vi "Create All Message Queues.vi"(8 "error in (no error)":errorcluster) -> (0 "error out":errorcluster, 3 "Message Queues out":T1)   [LabVIEW 2021, in "Message Queue.lvlib"]
doc: "This VI creates and initializes all the message queues for your application. If your application requires more than one message queue, right-click the \"Message Queues\" constant above and select Open Type Def. Add the new Message Queue(s) to the type definition, then initialize them in this VI."
uses:
  Message Queue.lvlib
  All Message Queues.ctl
  Message Cluster.ctl
  Enqueue Message (Single).vi
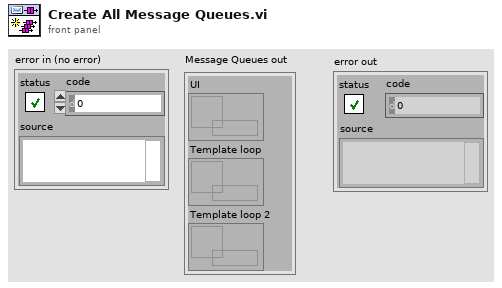
[diagram p1: front panel]
types:
  T1 = typedef "Message Queue.lvlib/All Message Queues.ctl" = cluster{"UI":refnum<queue>, "Template loop":refnum<queue>, "Template loop 2":refnum<queue>}
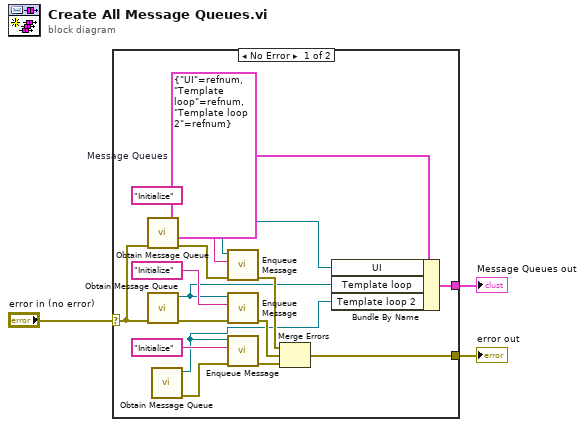
[diagram p0: block diagram]
diagram:
  n1 = case shown="No Error" "error in (no error)" {
    selector: "error in (no error)" -> [w8 w20]
    tunnel: [w10 w20] -> w3
    tunnel: [w18 _] -> w2
    frame No Error {
      w12 = T1 {"UI"=refnum, "Template loop"=refnum, "Template loop 2"=refnum}  # Message Queues
      n2 = call "Obtain Message Queue.vi"("error in (no error)"=w8) -> ("error out"=w17:errorcluster, "Message Queue"=w15:refnum<queue>)  [unwired: 9 in]
      n3 = call "Obtain Message Queue.vi"("error in (no error)"=w8) -> ("error out"=w14:errorcluster, "Message Queue"=w11:refnum<queue>)  [unwired: 9 in]
      n4 = call "Obtain Message Queue.vi"() -> ("error out"=w7:errorcluster, "Message Queue"=w4:refnum<queue>)  [unwired: 10 in]
      n5 = call-poly "Enqueue Message.vi"("error in (no error)"=w17, "Message"="Initialize", "Message Queue"=w15) -> ("error out"=w19:errorcluster)  [unwired: 7 in, 1 out]
      n6 = call-poly "Enqueue Message.vi"("error in (no error)"=w14, "Message"="Initialize", "Message Queue"=w11) -> ("error out"=w9:errorcluster)  [unwired: 7 in, 1 out]
      n7 = call-poly "Enqueue Message.vi"("error in (no error)"=w7, "Message"="Initialize", "Message Queue"=w4) -> ("error out"=w5:errorcluster)  [unwired: 7 in, 1 out]
      n8 = Merge Errors(w19, w9, w5) -> (w10:errorcluster)
      n9 = Bundle By Name(cluster=w12, "UI"=w15, "Template loop"=w11, "Template loop 2"=w4) -> (w18:T1)
    }
    frame Error {
    }
  }
  "Message Queues out" <- w2
  "error out" <- w3
